vi "Write Glyphs to  File.vi"(6 "File Name":string="Glyphs.bin", 7 "Path":T1=enum."Glyphs", 8 "error in (no error)":errorcluster, 11 "Graphics []":T2[](array[typedef])) -> (0 "error out":errorcluster)   [LabVIEW 2021]
uses:
  Controls/Path&Icon.ctl
  vi.lib/LabVIEW Icon API/lv_icon/Controls/Pathes.ctl
  vi.lib/LabVIEW Icon API/lv_icon/lv_icon.lvlib
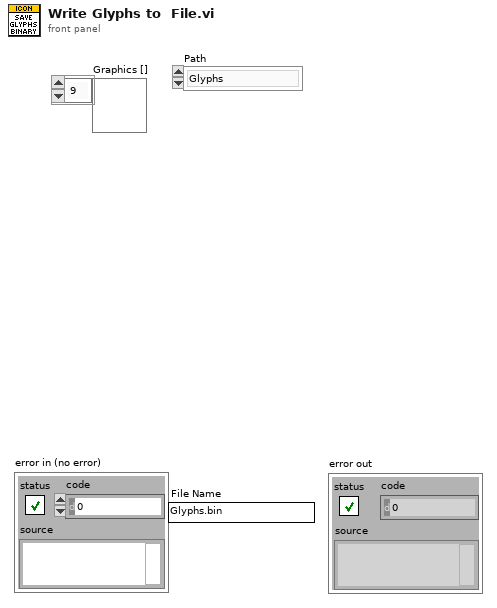
[diagram p1: front panel]
types:
  T1 = typedef "Pathes.ctl" = enum16{"Root Path", "Icon Templates", "Icon Templates VI", "Icon Templates Lib", "Glyphs"}
  T2 = typedef "Path&Icon.ctl" = cluster{"Rectangle":cluster{"left":i16, "top":i16, "right":i16, "bottom":i16}, "Path":path, "Image":picture, "Filter":string, "FileName":string}
  T3 = enum16{"open", "replace", "create", "open or create", "replace or create", "replace or create with confirmation"}
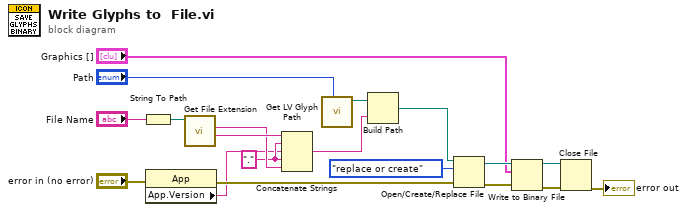
[diagram p0: block diagram]
diagram:
  w4 = "." ("string")
  n1 = String To Path(string="File Name") -> (path=w7:path)
  n2 = property class="App"(error in="error in (no error)") -> (error out=w10:errorcluster, "App.Version"=w1:string)  [unwired: 1 in, 1 out]
  n3 = call <vilib>:"Get File Extension.vi"("file"=w7) -> ("filename without extension"=w6:string, "lowercase file extension"=w5:string)  [unwired: 1 in, 8 out]
  n4 = Concatenate Strings(w6, w4, w1, w4, w5) -> (w2:string)
  n5 = call "Get LV Glyph Path.vi"("Path"="Path") -> ("Requested Path"=w18:path)  [unwired: 2 in, 8 out]
  n6 = Build Path(base path=w18, name or relative path=w2) -> (appended path=w9:path)
  n7 = Open/Create/Replace File(file path (use dialog)=w9, error in=w10, operation (0:open)=T3."replace or create") -> (refnum out=w16:refnum<file>, error out=w15:errorcluster)  [unwired: 1 in, 3 out]
  n8 = Write to Binary File(file (use dialog)=w16, data="Graphics []", error in=w15) -> (refnum out=w13:refnum<file>, error out=w14:errorcluster)  [unwired: 4 out]
  n9 = Close File(refnum=w13, error in=w14) -> (error out=→"error out":errorcluster)  [unwired: 1 out]
